vi "题目6.vi"   [LabVIEW 2017]
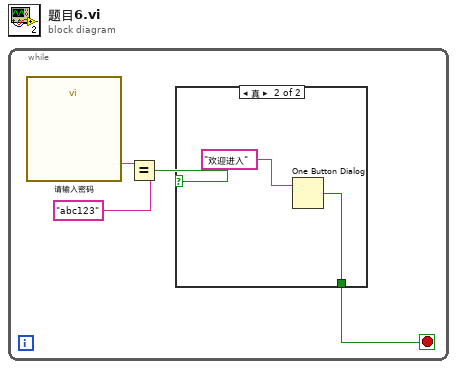
[diagram p0: block diagram]
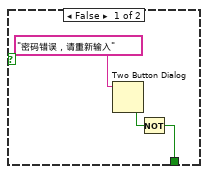
[diagram p2: hidden frame]
diagram:
  n1 = while {
    stop <- w1 stop-if-true
    n2 = call "请输入密码"() -> ("密码"=w2:string)  [unwired: 17 in, 2 out]
    n3 = Equal?(x=w2, y="abc123") -> (x = y?=w3:bool)
    n4 = case shown="真" w3 {
      tunnel: [w5 w8] -> w1
      frame False {
        n5 = Two Button Dialog(message="密码错误，请重新输入" ("消息")) -> (T button?=w6:bool)  [unwired: 2 in]
        n6 = Not(x=w6) -> (.not. x?=w5:bool)
      }
      frame True {
        n7 = One Button Dialog(message="欢迎进入" ("消息")) -> (true=w8:bool)  [unwired: 1 in]
      }
    }
  }
